vi "Modify_Image_Histogram-3.vi"(4 "[IN] Parameter":sgl format="%.2f", 6 "[IN] Operator":T4(ring), 7 "1 - Origin\n2 - LoG":u8, 8 "error IN":errorcluster, 9 "[IN] Image Filtering Settings":T1, 11 "[IN] LoG Processed Image":T3) -> (0 "error OUT":errorcluster, 1 "[OUT] Image Filtering Settings":T1, 2 "[OUT] Histogram":T2 {"Incremental Value" format="%.2f"; "Starting Value" format="%.2f"}, 3 "[OUT] Histogram Modified Image":T3)   [LabVIEW 2013]
doc: "This subVI modifies image through various mathlookup operations (see the built-in function \"IMAQ MathLookup\")\nThis subVI modifies image through various mathlookup operations (see the built-in function \"IMAQ MathLookup\")\nIn other words, it makes the gamma correction of picture (exchanging if intensity for each single pixel by multiplying of this pixel value on some function)"
uses:
  <vilib>/vision/Image Controls.llb/IMAQ Image.ctl
  <vilib>/vision/NI_Vision_Development_Module.lvlib
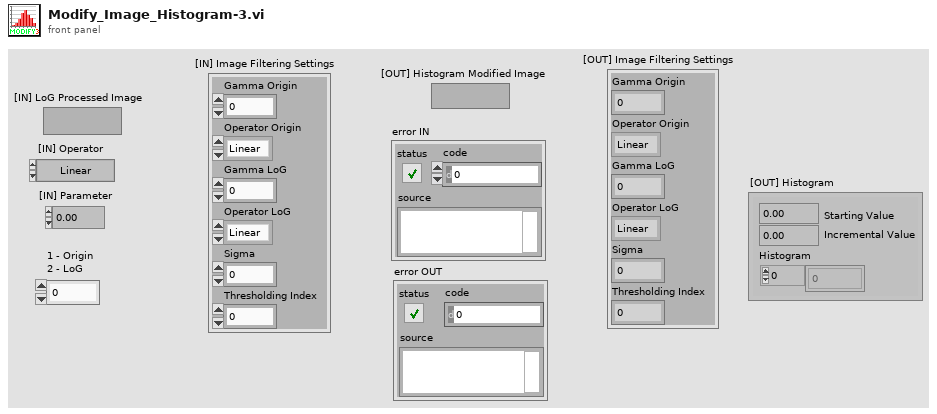
[diagram p1: front panel]
types:
  T1 = cluster{"Gamma Origin":sgl, "Operator Origin":enum32{"Linear", "Log", "Exp", "Square", "Square root", "Power X", "Power 1/X"}, "Gamma LoG":sgl, "Operator LoG":enum32{"Linear", "Log", "Exp", "Square", "Square root", "Power X", "Power 1/X"}, "Sigma":dbl, "Thresholding Index":i8}
  T2 = cluster{"Starting Value":sgl, "Incremental Value":sgl, "Histogram":u32[]}
  T3 = typedef "IMAQ Image.ctl" = refnum<image>
  T4 = enum32{"Linear", "Log", "Exp", "Square", "Square root", "Power X", "Power 1/X"}
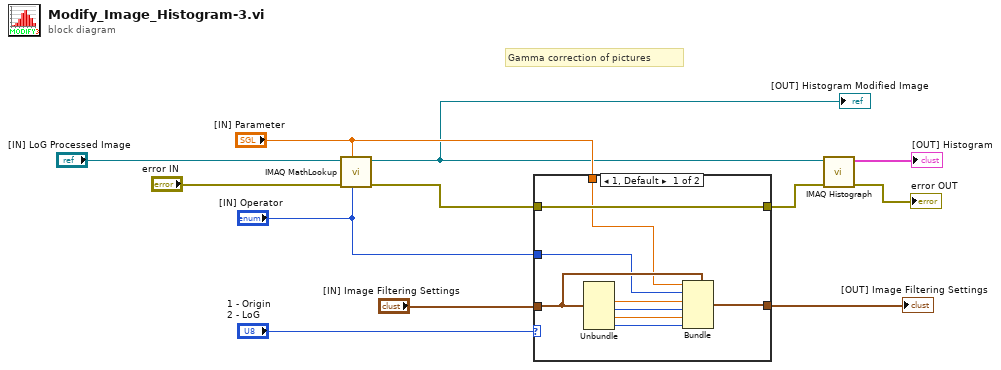
[diagram p0: block diagram]
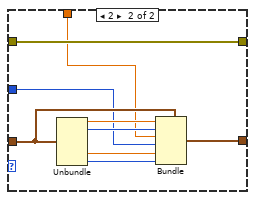
[diagram p2: hidden frame]
diagram:
  # "Gamma correction of pictures"
  n1 = call "IMAQ MathLookup"("Operator"="[IN] Operator", "X Value"="[IN] Parameter", "error in (no error)"="error IN", "Image Src"="[IN] LoG Processed Image") -> ("error out"=w6:errorcluster, "Image Dst Out"=w7:T3)  [unwired: 6 in]
  "[OUT] Histogram Modified Image" <- w7
  n2 = case shown="1, Default" "1 - Origin\n2 - LoG" {
    tunnel: "[IN] Parameter" -> [w14 w24]
    tunnel: "[IN] Operator" -> [w13 w23]
    tunnel: w6 -> [w21 w30]
    tunnel: [w21 w30] -> w5
    tunnel: "[IN] Image Filtering Settings" -> [w18 w29]
    tunnel: [w17 w22] -> w1
    frame 1, Default {
      n3 = Unbundle(w18) -> ("Gamma LoG"=w16:sgl, "Operator LoG"=w15:T4, "Sigma"=w19:dbl, "Thresholding Index"=w20:i8)  [unwired: 2 out]
      n4 = Bundle(cluster=w18, "Gamma Origin"=w14, "Operator Origin"=w13, "Gamma LoG"=w16, "Operator LoG"=w15, "Sigma"=w19, "Thresholding Index"=w20) -> (w17:T1)
    }
    frame 2 {
      n5 = Unbundle(w29) -> ("Gamma Origin"=w26:sgl, "Operator Origin"=w25:T4, "Sigma"=w27:dbl, "Thresholding Index"=w28:i8)  [unwired: 2 out]
      n6 = Bundle(cluster=w29, "Gamma Origin"=w26, "Operator Origin"=w25, "Gamma LoG"=w24, "Operator LoG"=w23, "Sigma"=w27, "Thresholding Index"=w28) -> (w22:T1)
    }
  }
  "[OUT] Image Filtering Settings" <- w1
  n7 = call "IMAQ Histograph"("error in (no error)"=w5, "Image"=w7) -> ("error out"=→"error OUT":errorcluster, "Histogram Graph"=→"[OUT] Histogram":T2)  [unwired: 6 in, 2 out]
